vi "Show Window.vi"(4 "error in (no error)":errorcluster, 6 "window name (\"\")":string, 7 "window refnum (NaWR)":T1) -> (0 "error out":errorcluster, 3 "window refnum out":T1)   [LabVIEW 2023, in "WINUTIL.lvlib"]
doc: "This function will show a previously hidden window. The window named in the 'window name' input is used to identify the target window if 'window refnum' is invalid. If the window cannot be found, an error will be returned and 'window refnum out' will be invalid."
uses:
  WINUTIL.lvlib
  Window Refnum.ctl
  LVWUtil32.dll
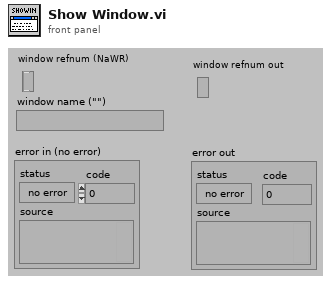
[diagram p1: front panel]
types:
  T1 = typedef "WINUTIL.lvlib/Window Refnum.ctl" = refnum<k1>
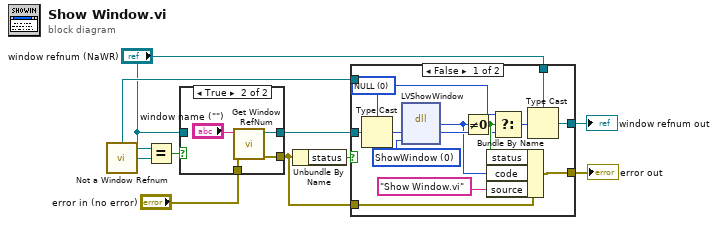
[diagram p0: block diagram]
diagram:
  n1 = call "Not a Window Refnum.vi"() -> ("Not a Window Refnum"=w4:T1)
  n2 = Equal?(x="window refnum (NaWR)", y=w4) -> (x = y?=w5:bool)
  n3 = case shown="True" w5 {
    tunnel: "error in (no error)" -> [w10 w15]
    tunnel: [w11 w14] -> w2
    tunnel: "window refnum (NaWR)" -> [w11 _]
    tunnel: [w10 w13] -> w8
    frame False {
    }
    frame True {
      n4 = call "Get Window RefNum.vi"("error in (no error)"=w15, "window name (\"\")"="window name (\"\")") -> ("error out"=w13:errorcluster, "window refnum (NaWR)"=w14:T1)  [unwired: 6 out]
    }
  }
  n5 = Unbundle By Name(w8) -> ("status"=w9:bool)
  n6 = case shown="False" w9 {
    tunnel: w8 -> [w24 w30]
    tunnel: [w28 w30] -> w6
    tunnel: w2 -> [w22 _]
    tunnel: [w21 w29] -> w1
    tunnel: "window refnum (NaWR)" -> [w20 _]
    tunnel: w4 -> [_ w29]
    frame False {
      w19 = u8 0 items=["ShowWindow"]
      w23 = u32 0 items=["NULL"]
      n7 = Type Cast(type=w23, x=w22) -> (*(type *) &x=w16:u32)
      n8 = dll-call lib="C:/Users/acasalen/Documents/LabVIEW Data/Projects/Reds-Auto-Clicker/Red's Auto Clicker/SubVIs/labview_win_util32_8.6/lvwutil32.dll" fn="LVShowWindow"("hWnd"=w16, "function"=w19) -> ("error"=w17:i32, "hWnd"=w18:u32)  [unwired: 4 in, 2 out]
      n9 = Not Equal To 0?(x=w17) -> (x != 0?=w26:bool)
      n10 = Bundle By Name(cluster=w24, "status"=w26, "code"=w17, "source"="Show Window.vi") -> (w28:errorcluster)
      n11 = Select(t=w23, s=w26, f=w18) -> (s? t:f=w27:u32)
      n12 = Type Cast(type=w20, x=w27) -> (*(type *) &x=w21:T1)
    }
    frame True {
    }
  }
  "error out" <- w6
  "window refnum out" <- w1
